vi "Read (Measurement).vi"(7 "Measurement (0:Frequency)":i32(ring) items=["Frequency", "Frequency Ratio", "Period", "Totalize", "Phase", "Edge Rise Time", "Edge Fall Time", "Positive Pulse Width", "Negative Pulse Width", "Duty Cycle", "Time Interval", "Volt Maximum", "Volt Minimum"], 8 "error in (no error)":errorcluster, 9 "Maximum Time (10000 ms)":u32=10000, 11 "VISA resource name":refnum<visa-resource-name>) -> (0 "error out":errorcluster, 2 "Measurement":dbl format="%#.10g", 3 "VISA resource name out":refnum<visa-resource-name>)   [LabVIEW 2020, in "Counter.lvlib" / "PICOTEST U62XXA series.lvlib"]
doc: "Reads and returns a single Measurement.\n\n<B>Note:</B>\n\nIf no valid result exists, Not a Number 9.91E37 is returned."
uses:
  PICOTEST U62XXA series.lvlib
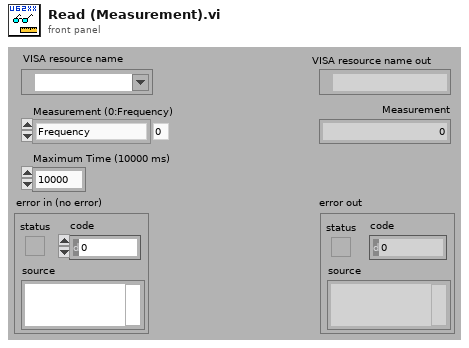
[diagram p1: front panel]
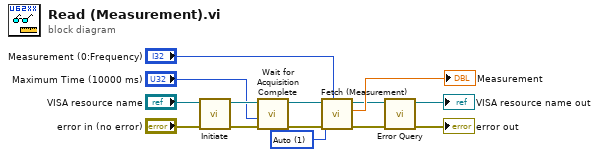
[diagram p0: block diagram]
diagram:
  w1 = 1 items=["Time/External", "Auto"] ("Totalize Arm Type (0:Time/External)")
  n1 = call "Initiate.vi"("error in (no error)"="error in (no error)", "VISA resource name"="VISA resource name") -> ("error out"=w6:errorcluster, "VISA resource name out"=w7:refnum<visa-resource-name>)  [unwired: 8 in]
  n2 = call "Wait for Acquisition Complete.vi"("error in (no error)"=w6, "Maximum Time (10000 ms)"="Maximum Time (10000 ms)", "VISA resource name"=w7) -> ("error out"=w4:errorcluster, "VISA resource name out"=w5:refnum<visa-resource-name>)  [unwired: 7 in]
  n3 = call "Fetch (Measurement).vi"("Measurement (0:Frequency)"="Measurement (0:Frequency)", "error in (no error)"=w4, "Totalize Arm Type (0:Time/External)"=w1, "VISA resource name"=w5) -> ("error out"=w10:errorcluster, "Result"=→"Measurement":dbl, "VISA resource name out"=w11:refnum<visa-resource-name>)  [unwired: 5 in]
  n4 = call "Error Query.vi"("error in (no error)"=w10, "VISA resource name"=w11) -> ("error out"=→"error out":errorcluster, "VISA resource name out"=→"VISA resource name out":refnum<visa-resource-name>)  [unwired: 6 in, 2 out]
